vi "Re-tag Larvae (SubVI).vi"(0 "Image Size":T2={"Height"=512, "Width"=512} {"Width" step=8; "Height" step=8}, 1 "BG SUB TH":i16=20, 2 "Subtract BG":bool, 3 "BG Image":u8[][](array[numeric]), 5 "Data In":T1, 6 "Range":cluster{"Lower value":u8, "Upper value":u8}={"Lower value"=100, "Upper value"=255}, 7 "Min Distance":sgl=100.0, 8 "Box Side":cluster{"Low":u32, "High":u32}={"Low"=16, "High"=96}, 10 "Box W + L":cluster{"Low":u32, "High":u32}={"Low"=40, "High"=150}, 12 "Area":cluster{"Low":u32, "High":u32}={"Low"=448, "High"=1280}) -> (14 "# of Objects":i32, 16 "BBOX Array":u64[](array[numeric]), 19 "HT LOC":u64[](array[numeric]))   [LabVIEW 2015]
uses:
  Controls (HOST)/Image Size.ctl
  Controls (HOST)/Data to Disk Bundle.ctl
  <vilib>/vision/NI_Vision_Development_Module.lvlib
panel:
  out "cHy":u16[](array[numeric])
  out "cHx":u16[](array[numeric])
  out "cTy":u16[](array[numeric])
  out "cTx":u16[](array[numeric])
  out "pHy":u16[](array[numeric])
  out "pHx":u16[](array[numeric])
  out "pTy":u16[](array[numeric])
  out "pTx":u16[](array[numeric])
  out "HT Found?":bool[](array[boolean])
  out "HT Distance":sgl[](array[numeric])
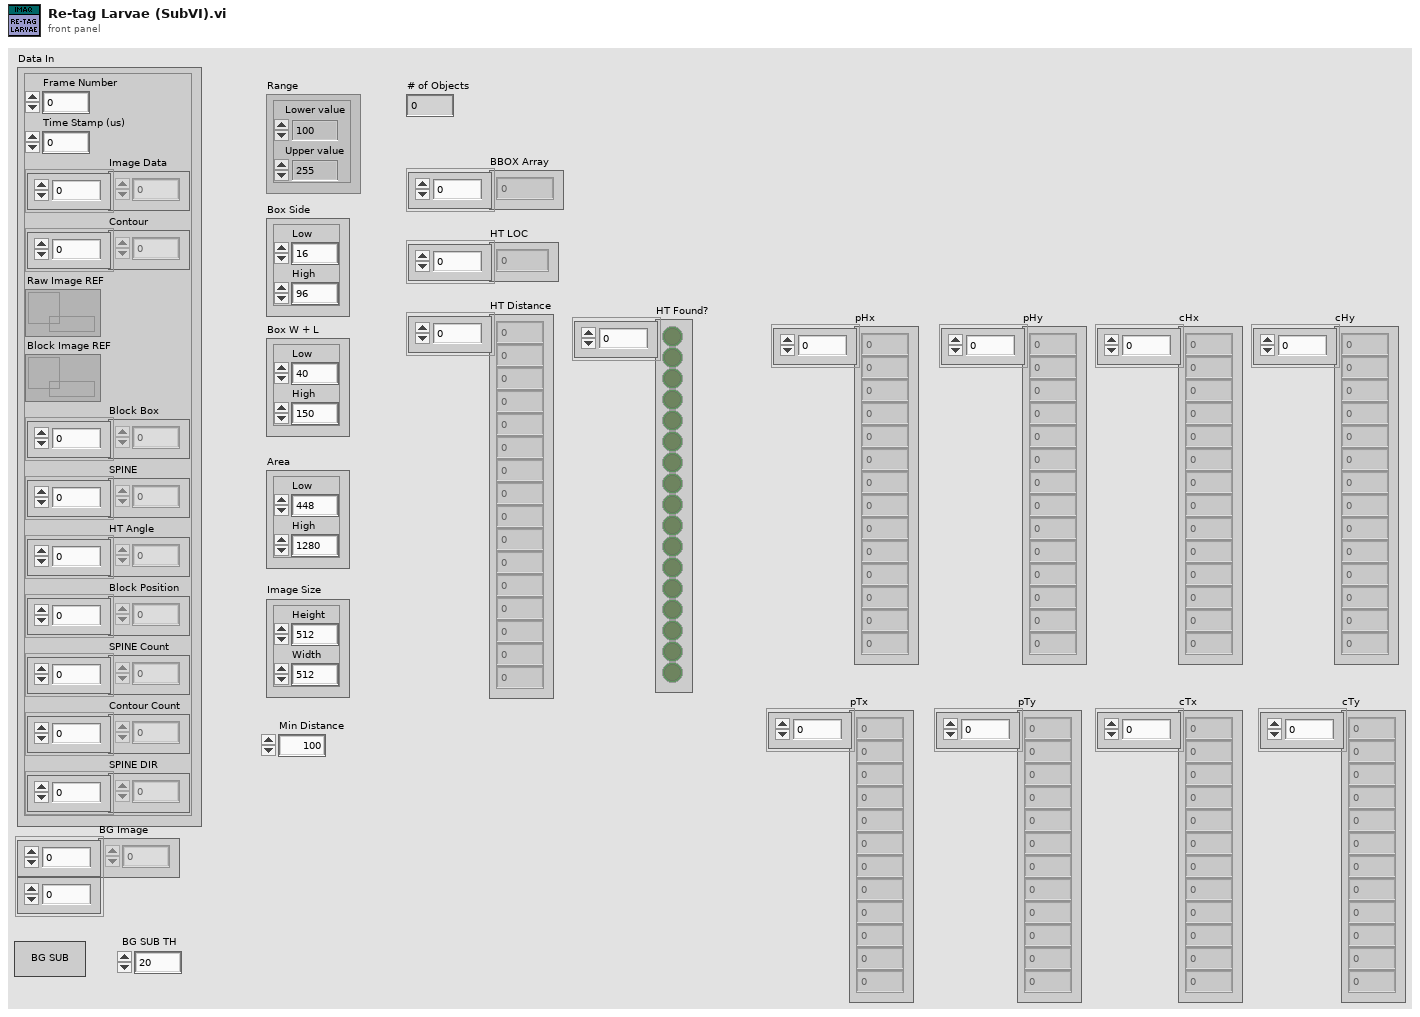
[diagram p1: front panel]
types:
  T1 = typedef "Data to Disk Bundle.ctl" = cluster{"Frame Number":u64, "Time Stamp (us)":u64, "Image Data":u64[], "Contour":u32[], "Raw Image REF":refnum<data-value>, "Block Image REF":refnum<data-value>, "Block Box":u64[], "SPINE":u32[], "HT Angle":u64[], "Block Position":u64[], "SPINE Count":u32[], "Contour Count":u32[], "SPINE DIR":u8[]}
  T2 = typedef "Image Size.ctl" = cluster{"Height":u16, "Width":u16}
  T3 = enum16{"big-endian, network order", "native, host order", "little-endian"}
  T4 = typedef "IMAQ Image.ctl" = refnum<image>
  T5 = cluster{"Area":dbl, "Number of Holes":dbl, "Bounding Rect":cluster{"Left":dbl, "Top":dbl, "Right":dbl, "Bottom":dbl}, "Center of Mass":cluster{"X":dbl, "Y":dbl}, "Orientation":dbl, "Dimensions":cluster{"Width":dbl, "Height":dbl}}[]
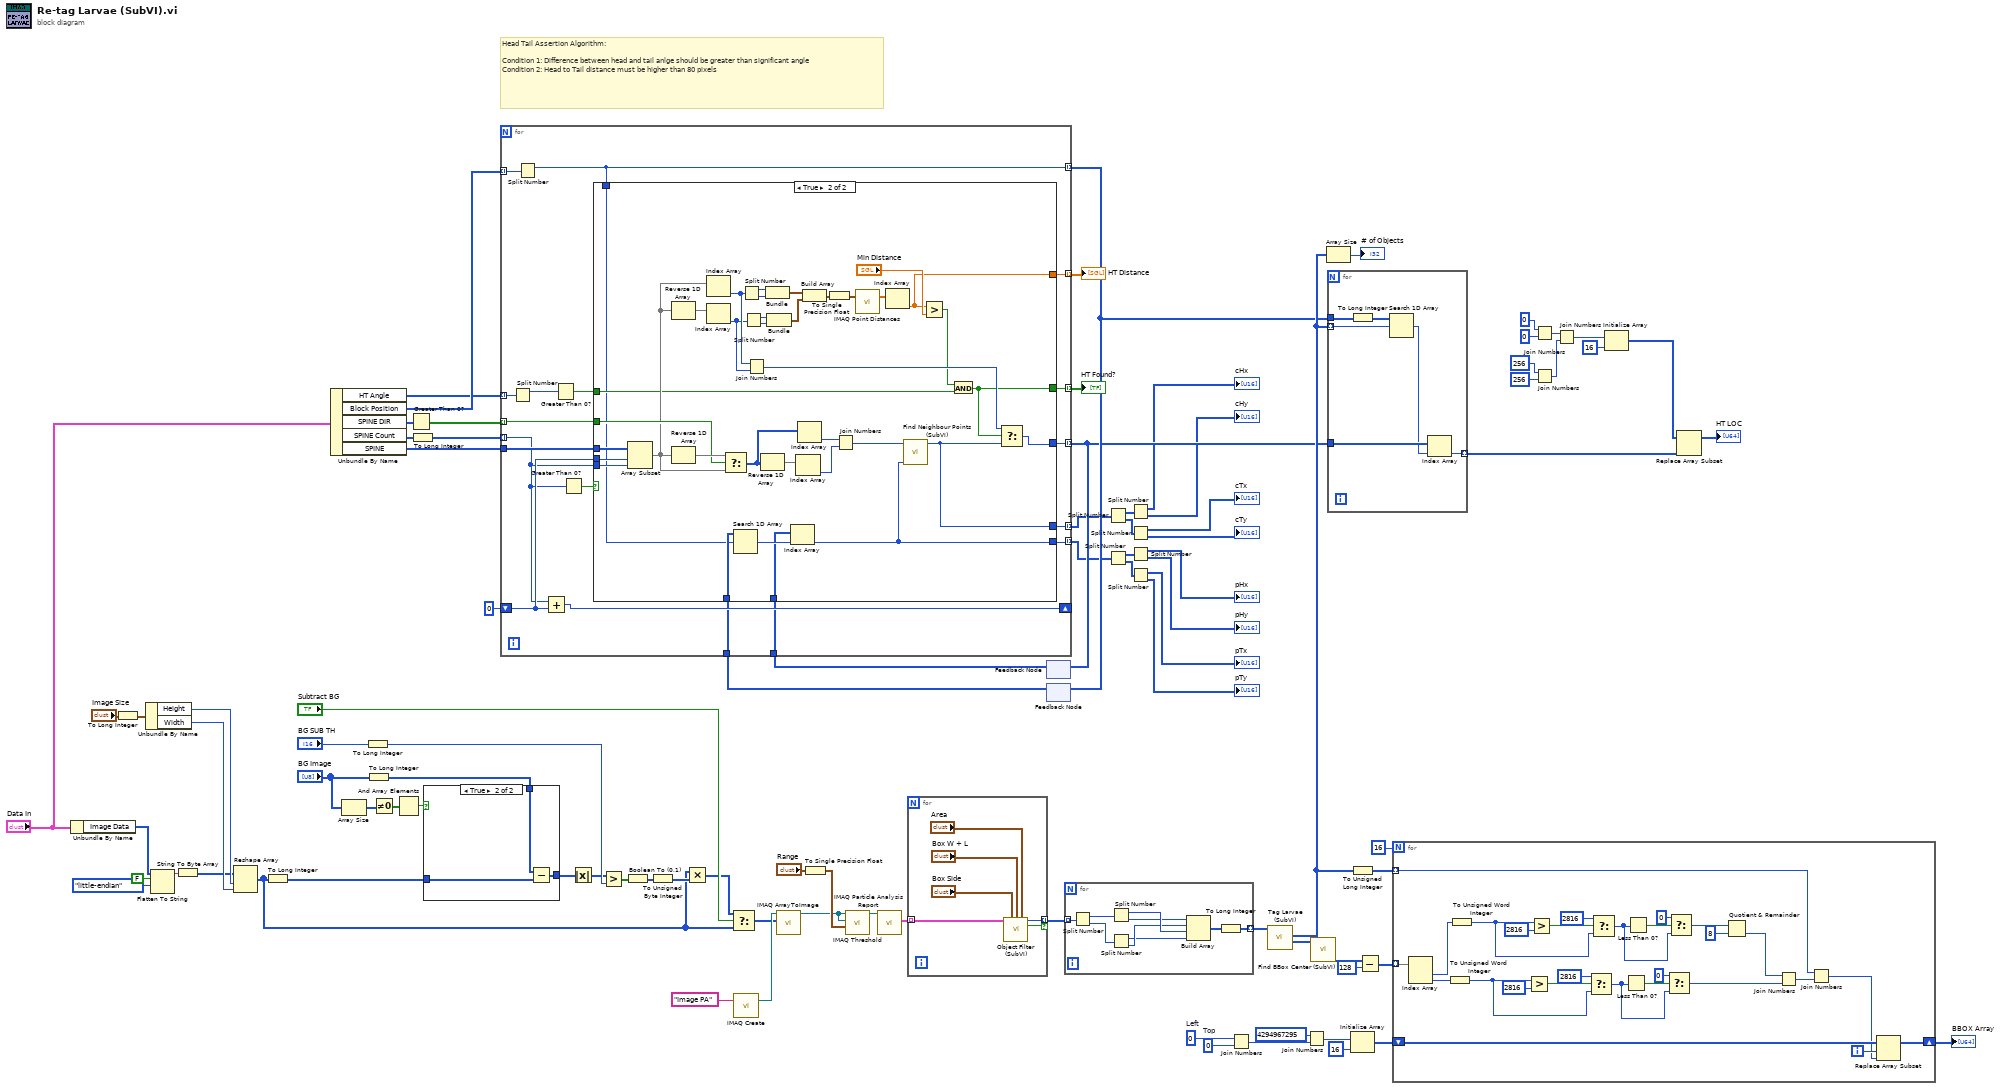
[diagram p0: block diagram]
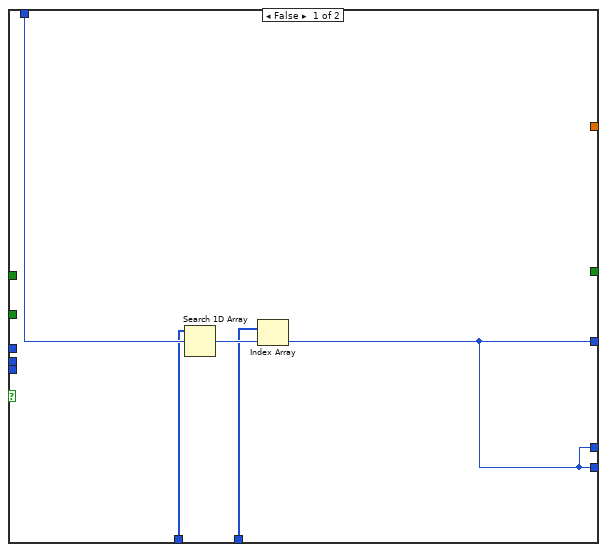
[diagram p2: hidden frame]
diagram:
  w74 = u16 0  # Left
  w70 = u16 0  # Top
  # "Head Tail Assertion Algorithm:\n\nCondition 1: Difference between head and tail anlge should be greater than significant angle\nCondition 2: Head to Tail distance must be higher than 80 pixels"
  n1 = Unbundle By Name("Data In") -> ("Image Data"=w57:u64[])
  n2 = To Long Integer(number="Image Size") -> (32bit integer=w50:cluster{"Height":i32, "Width":i32})
  n3 = Unbundle By Name(w50) -> ("Height"=w52:i32, "Width"=w51:i32)
  n4 = Flatten To String(anything=w57, prepend array or string size? (T)=FALSE, byte order (0:big-endian, network order)=T3."little-endian") -> (data string=w54:string)  [unwired: 1 in, 2 out]
  n5 = String To Byte Array(string=w54) -> (unsigned byte array=w44:u8[])
  n6 = Reshape Array(w44, w52, w51) -> (w18:u8[][])
  n7 = To Long Integer(number=w18) -> (32bit integer=w67:i32[][])
  n8 = Unbundle By Name("Data In") -> ("HT Angle"=w17:u64[], "Block Position"=w35:u64[], "SPINE DIR"=w38:u8[], "SPINE Count"=w42:u32[], "SPINE"=w41:u32[])
  n9 = Array Size(array="BG Image") -> (size(s)=w47:i32[])
  n10 = To Long Integer(number="BG SUB TH") -> (32bit integer=w58:i32)
  n11 = To Long Integer(number="BG Image") -> (32bit integer=w66:i32[][])
  n12 = Not Equal To 0?(x=w47) -> (x != 0?=w46:bool[])
  n13 = And Array Elements(Boolean array=w46) -> (logical AND=w45:bool)
  n14 = Greater Than 0?(x=w38) -> (x > 0?=w37:bool[])
  n15 = To Long Integer(number=w42) -> (32bit integer=w39:i32[])
  n16 = case shown="True" w45 {
    tunnel: w67 -> [w92 w95]
    tunnel: w66 -> [_ w94]
    tunnel: [w92 w93] -> w65
    frame False {
    }
    frame True {
      n17 = Subtract(x=w94, y=w95) -> (x-y=w93:i32[][])
    }
  }
  n18 = Absolute Value(x=w65) -> (abs(x)=w43:i32[][])
  n19 = Greater?(x=w43, y=w58) -> (0:w63:bool[][])
  n20 = Boolean To (0,1)(Boolean=w63) -> (0, 1=w62:i16[][])
  n21 = To Unsigned Byte Integer(number=w62) -> (unsigned 8bit integer=w61:u8[][])
  n22 = Multiply(x=w18, y=w61) -> (x*y=w60:u8[][])
  n23 = Select(t=w60, s="Subtract BG", f=w18) -> (s? t:f=w49:u8[][])
  n24 = call "IMAQ Create"("Image Name"="Image PA") -> ("New Image"=w83:T4)  [unwired: 4 in, 1 out]
  n25 = call "IMAQ ArrayToImage"("Image Pixels (U8)"=w49, "Image"=w83) -> ("Image Out"=w85:T4)  [unwired: 8 in, 1 out]
  n26 = To Single Precision Float(number="Range") -> (single precision float=w91:cluster{"Lower value":sgl, "Upper value":sgl})
  n27 = call "IMAQ Threshold"("Range"=w91, "Image Dst"=w85, "Image Src"=w85) -> ("Image Dst Out"=w84:T4)  [unwired: 7 in, 1 out]
  n28 = call "IMAQ Particle Analysis Report"("Image"=w84) -> ("Particle Reports (Pixels)"=w87:T5)  [unwired: 5 in, 5 out]
  n29 = for {
    tunnel: w87 -> [w97] mode=indexing
    tunnel: [w101] -> w88 mode=indexing if=w96
    n30 = call "Object Filter (SubVI).vi"("Particle Report"=w97, "Box Side"="Box Side", "Box W + L"="Box W + L", "Area"="Area") -> ("Bounding Box"=w101:u64, "Data Valid"=w96:bool)  [unwired: 10 in]
  }
  n31 = feedback #1() -> (w20:u64[])  [unwired: 1 in]
  n32 = feedback #2() -> (w22:u32[])  [unwired: 1 in]
  n33 = for {
    tunnel: w39 -> [w112] mode=indexing
    tunnel: w41 -> [w118]
    shift-right: [w119] -> _
    shift-left: 0 ("Numeric Control") -> [w117]
    tunnel: w37 -> [w116] mode=indexing
    tunnel: [w115] -> w21 mode=indexing
    tunnel: w35 -> [w114] mode=indexing
    tunnel: [w111] -> w23 mode=indexing
    tunnel: w22 -> [w110]
    tunnel: w20 -> [w109]
    tunnel: w17 -> [w108] mode=indexing
    tunnel: [w105] -> w16 mode=indexing
    tunnel: [w104] -> w15 mode=indexing
    tunnel: [w103] -> w14 mode=indexing
    tunnel: [w102] -> w13 mode=indexing
    n34 = Split Number(x=w108) -> (hi(x)=w107:u32)  [unwired: 1 out]
    n35 = Split Number(x=w114) -> (hi(x)=w111:u32)  [unwired: 1 out]
    n36 = Add(x=w112, y=w117) -> (x+y=w119:i32)
    n37 = Greater Than 0?(x=w107) -> (x > 0?=w106:bool)
    n38 = Greater Than 0?(x=w112) -> (x > 0?=w113:bool)
    n39 = case shown="True" w113 {
      tunnel: w118 -> [_ w160]
      tunnel: w112 -> [_ w159]
      tunnel: w117 -> [_ w158]
      tunnel: w116 -> [_ w155]
      tunnel: [w120 w139] -> w115
      tunnel: w111 -> [w124 w131]
      tunnel: w110 -> [w123 w133]
      tunnel: w109 -> [w121 w132]
      tunnel: w106 -> [_ w136]
      tunnel: [_ w135] -> w105
      tunnel: [_ w127] -> w104
      tunnel: [w120 w126] -> w103
      tunnel: [w120 w125] -> w102
      frame False {
        n40 = Search 1D Array(1D array=w123, element=w124) -> (index of element=w122:i32)  [unwired: 1 in]
        n41 = Index Array(array=w121, index=w122) -> (element=w120:u64)
      }
      frame True {
        n42 = Array Subset(array=w160, index=w158, length=w159) -> (w152:u32[])
        n43 = Reverse 1D Array(array=w152) -> (reversed array=w153:u32[])
        n44 = Reverse 1D Array(array=w152) -> (reversed array=w157:u32[])
        n45 = Index Array(array=w152) -> (element=w141:u32)  [unwired: 1 in]
        n46 = Index Array(array=w153) -> (element=w140:u32)  [unwired: 1 in]
        n47 = Select(t=w157, s=w155, f=w152) -> (s? t:f=w154:u32[])
        n48 = Search 1D Array(1D array=w133, element=w131) -> (index of element=w134:i32)  [unwired: 1 in]
        n49 = Split Number(x=w141) -> (hi(x)=w151:u16, lo(x)=w148:u16)
        n50 = Split Number(x=w140) -> (hi(x)=w149:u16, lo(x)=w150:u16)
        n51 = Join Numbers(hi=w141, lo=w140) -> ((hi.lo)=w138:u64)
        n52 = Reverse 1D Array(array=w154) -> (reversed array=w156:u32[])
        n53 = Bundle(w151, w148) -> (w147:cluster{u16, u16})  [unwired: 1 in]
        n54 = Bundle(w149, w150) -> (w146:cluster{u16, u16})  [unwired: 1 in]
        n55 = Index Array(array=w132, index=w134) -> (element=w126:u64)
        n56 = Index Array(array=w156) -> (element=w129:u32)  [unwired: 1 in]
        n57 = Index Array(array=w154) -> (element=w128:u32)  [unwired: 1 in]
        n58 = Build Array(w147, w146) -> (w145:cluster{u16, u16}[])
        n59 = To Single Precision Float(number=w145) -> (single precision float=w144:cluster{sgl, sgl}[])
        n60 = Join Numbers(hi=w128, lo=w129) -> ((hi.lo)=w130:u64)
        n61 = call "IMAQ Point Distances"("Points"=w144) -> ("Distances"=w143:sgl[])  [unwired: 4 in, 1 out]
        n62 = Index Array(array=w143) -> (element=w135:sgl)  [unwired: 1 in]
        n63 = call "Find Neighbour Points (SubVI).vi"("Previous HT Position"=w126, "Current HT Position"=w130) -> ("Neighbor Point"=w125:u64)  [unwired: 8 in, 1 out]
        n64 = Greater?(x=w135, y="Min Distance") -> (0:w137:bool)
        n65 = And(x=w137, y=w136) -> (x .and. y?=w127:bool)
        n66 = Select(t=w138, s=w127, f=w125) -> (s? t:f=w139:u64)
      }
    }
  }
  "HT Distance" <- w16
  "HT Found?" <- w15
  n67 = feedback-in #1(w21) -> ()
  n68 = feedback-in #2(w23) -> ()
  n69 = for {
    tunnel: w88 -> [w169] mode=indexing
    tunnel: [w161] -> w68 mode=indexing
    n70 = Split Number(x=w169) -> (hi(x)=w168:u32, lo(x)=w167:u32)
    n71 = Split Number(x=w168) -> (hi(x)=w166:u16, lo(x)=w165:u16)
    n72 = Split Number(x=w167) -> (hi(x)=w163:u16, lo(x)=w164:u16)
    n73 = Build Array(w165, w164, w166, w163) -> (w162:u16[])
    n74 = To Long Integer(number=w162) -> (32bit integer=w161:i32[])
  }
  n75 = Split Number(x=w13) -> (hi(x)=w12:u32[], lo(x)=w11:u32[])
  n76 = Split Number(x=w14) -> (hi(x)=w10:u32[], lo(x)=w9:u32[])
  n77 = Split Number(x=w12) -> (hi(x)=→"cHx":u16[], lo(x)=→"cHy":u16[])
  n78 = Split Number(x=w11) -> (hi(x)=→"cTx":u16[], lo(x)=→"cTy":u16[])
  n79 = Split Number(x=w10) -> (hi(x)=→"pHx":u16[], lo(x)=→"pHy":u16[])
  n80 = Split Number(x=w9) -> (hi(x)=→"pTx":u16[], lo(x)=→"pTy":u16[])
  n81 = Join Numbers(hi=w74, lo=w70) -> ((hi.lo)=w71:u32)
  n82 = call "Tag Larvae (SubVI).vi"("Array in"=w68) -> ("Bounding Box"=w77:i32[][], "Current ID"=w34:i32[])  [unwired: 8 in, 1 out]
  n83 = Join Numbers(hi=u32 4294967295, lo=w71) -> ((hi.lo)=w72:u64)
  n84 = call "Find BBox Center (SubVI).vi"("BBox Array In"=w77) -> ("Center Array"=w78:i32[][])  [unwired: 9 in, 1 out]
  n85 = Array Size(array=w34) -> (size(s)=→"# of Objects":i32)
  n86 = for {
    tunnel: w34 -> [w174] mode=indexing
    tunnel: w23 -> [w175]
    tunnel: w21 -> [w172]
    tunnel: [w171] -> w25 mode=indexing
    n87 = To Long Integer(number=w175) -> (32bit integer=w173:i32[])
    n88 = Search 1D Array(1D array=w173, element=w174) -> (index of element=w170:i32)  [unwired: 1 in]
    n89 = Index Array(array=w172, index=w170) -> (element=w171:u64)
  }
  n90 = To Unsigned Long Integer(number=w34) -> (unsigned 32bit integer=w90:u32[])
  n91 = Initialize Array(w72, 16 ("dimension size")) -> (w75:u64[])
  n92 = Subtract(x=w78, y=128) -> (x-y=w79:i32[][])
  n93 = for {
    N: 16 -> [_]
    shift-right: [w201] -> w81
    shift-left: w75 -> [w202]
    tunnel: w79 -> [w199] mode=indexing
    tunnel: w90 -> [w177] mode=indexing
    i -> [w200]
    n94 = Index Array(array=w199) -> (element #1=w181:i32, element #2=w182:i32)  [unwired: 2 in]
    n95 = To Unsigned Word Integer(number=w182) -> (unsigned 16bit integer=w192:u16)
    n96 = To Unsigned Word Integer(number=w181) -> (unsigned 16bit integer=w191:u16)
    n97 = Greater?(x=w192, y=u16 2816) -> (0:w198:bool)
    n98 = Greater?(x=w191, y=u16 2816) -> (0:w185:bool)
    n99 = Select(t=u16 2816 ("y"), s=w198, f=w192) -> (s? t:f=w194:u16)
    n100 = Select(t=u16 2816 ("y"), s=w185, f=w191) -> (s? t:f=w189:u16)
    n101 = Less Than 0?(x=w194) -> (x < 0?=w195:bool)
    n102 = Less Than 0?(x=w189) -> (x < 0?=w188:bool)
    n103 = Select(t=u16 0 ("y"), s=w195, f=w194) -> (s? t:f=w179:u16)
    n104 = Select(t=u16 0 ("y"), s=w188, f=w189) -> (s? t:f=w184:u16)
    n105 = Quotient & Remainder(x=w184, y=u16 8) -> (floor(x/y)=w180:u16)  [unwired: 1 out]
    n106 = Join Numbers(hi=w180, lo=w179) -> ((hi.lo)=w178:u32)
    n107 = Join Numbers(hi=w177, lo=w178) -> ((hi.lo)=w176:u64)
    n108 = Replace Array Subset(array=w202, new element=w176, index=w200) -> (w201:u64[])
  }
  "BBOX Array" <- w81
  n109 = Join Numbers(hi=u16 0 ("Numeric Control"), lo=u16 0 ("Numeric Control")) -> ((hi.lo)=w29:u32)
  n110 = Join Numbers(hi=u16 256 ("Numeric Control"), lo=u16 256 ("Numeric Control")) -> ((hi.lo)=w28:u32)
  n111 = Join Numbers(hi=w29, lo=w28) -> ((hi.lo)=w27:u64)
  n112 = Initialize Array(w27, 16 ("dimension size")) -> (w19:u64[])
  n113 = Replace Array Subset(array=w19, new element=w25) -> (→"HT LOC":u64[])  [unwired: 1 in]
